vi "Configure DMM_4 wire Resistance.vi"(0 "Semiconductor Module Context":T1, 5 "Pins":string[](array[string])=["RF1"], 11 "Error In":errorcluster) -> (15 "Error Out":errorcluster)   [LabVIEW 2013]
uses:
  <vilib>/NI_TestStand_SemiconductorModule/NI_TestStand_Semiconductor_Module.lvlibp/PinMap/General/SemiconductorModuleContext.ctl
  <instrlib>/niDMM/nidmm.llb/niDMM Powerline Frequency.ctl
  <instrlib>/niDMM/nidmm.llb/niDMM Offset Comp Ohms.ctl
  <instrlib>/niDMM/nidmm.llb/niDMM Resolution in Digits.ctl
  <instrlib>/niDMM/nidmm.llb/niDMM Function.ctl
  <instrlib>/niDMM/nidmm.llb/niDMM Auto Zero.ctl
  <instrlib>/niDMM/nidmm.llb/niDMM Configure Measurement Digits.vi
  Pin Map API/DMM Custom Instruments.lvlib
  <vilib>/NI_TestStand_SemiconductorModule/NI_TestStand_Semiconductor_Module.lvlibp
panel:
  in  "Range":dbl=10.0 format="%.2p"
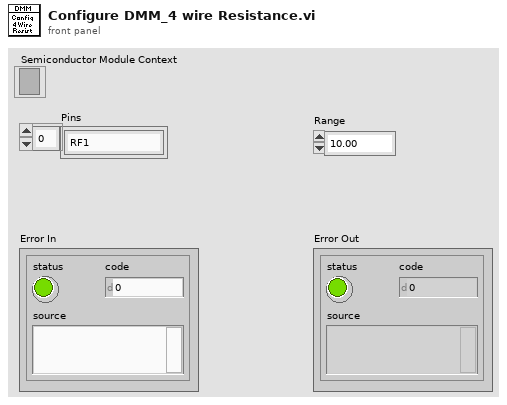
[diagram p1: front panel]
types:
  T1 = typedef "NI_TestStand_Semiconductor_Module.lvlibp/SemiconductorModuleContext.ctl" = refnum<k7>
  T2 = typedef "niDMM Function.ctl" = enum16{"DC Volts", "AC Volts", "DC Current", "AC Current", "2-wire Resistance", "4-wire Resistance", "Diode", "Frequency", "Period", "AC Volts DC Coupled", "Capacitance", "Inductance", "Temperature"}
  T3 = typedef "niDMM Powerline Frequency.ctl" = enum16{"60 Hz", "50 Hz"}
  T4 = typedef "niDMM Auto Zero.ctl" = i32
  T5 = typedef "niDMM Resolution in Digits.ctl" = dbl
  T6 = typedef "niDMM Offset Comp Ohms.ctl" = i32
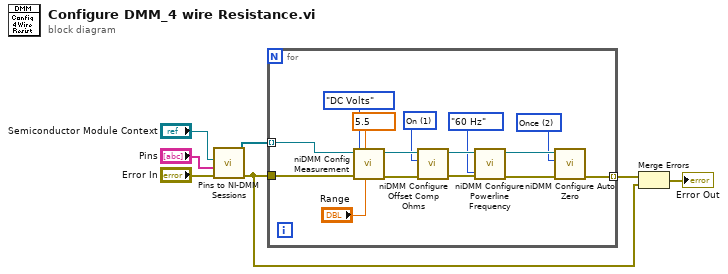
[diagram p0: block diagram]
diagram:
  n1 = call "Pins to NI-DMM Sessions.vi"("error in (no error)"="Error In", "Pins"="Pins", "Semiconductor Module Context"="Semiconductor Module Context") -> ("error out"=w6:errorcluster, "Instrument Sessions"=w7:refnum<k15>[])  [unwired: 4 in, 3 out]
  n2 = for {
    tunnel: w7 -> [w12] mode=indexing
    tunnel: w6 -> [w13]
    tunnel: [w10] -> w1 mode=indexing
    w8 = T4 2 items=["Auto"=-1, "Off"=0, "On"=1, "Once"=2] ("Auto Zero")
    w14 = T5 5.5 items=["3 1/2"=3.5, "4 1/2"=4.5, "5 1/2"=5.5, "6 1/2"=6.5, "7 1/2"=7.5] ("Resolution in Digits")
    w18 = T6 1 items=["Off", "On"] ("Offset Compensated Ohms")
    n3 = call-poly <instrlib>:"niDMM Config Measurement.vi"("Range"="Range", "Resolution in Digits"=w14, "error in (no error)"=w13, "Function"=niDMM_Function."DC Volts" ("Measurement Type"), "instrument handle"=w12) -> ("error out"=w20:errorcluster, "instrument handle out"=w19:refnum<k15>)  [unwired: 5 in]
    n4 = call <instrlib>:"niDMM Configure Offset Comp Ohms.vi"("error in (no error)"=w20, "Offset Compensated Ohms"=w18, "instrument handle"=w19) -> ("error out"=w17:errorcluster, "instrument handle out"=w16:refnum<k15>)  [unwired: 7 in]
    n5 = call <instrlib>:"niDMM Configure Powerline Frequency.vi"("Powerline Frequency"=niDMM_Powerline_Frequency."60 Hz", "error in (no error)"=w17, "instrument handle"=w16) -> ("error out"=w11:errorcluster, "instrument handle out"=w9:refnum<k15>)  [unwired: 7 in]
    n6 = call <instrlib>:"niDMM Configure Auto Zero.vi"("error in (no error)"=w11, "Auto Zero"=w8, "instrument handle"=w9) -> ("error out"=w10:errorcluster)  [unwired: 7 in, 1 out]
  }
  n7 = Merge Errors(w1, w6) -> (→"Error Out":errorcluster)
